vi "VelocityEstimator.vi"(8 "error in (no error)":errorcluster, 11 "Position In":dbl[](array[numeric])) -> (0 "error out":errorcluster, 3 "Vel. Out":dbl[](array[numeric]))   [LabVIEW 2018, in "Motor_ReadAng.lvlib"]
doc: "Estimate motor velocity from the motor position."
uses:
  Motor_ReadAng.lvlib
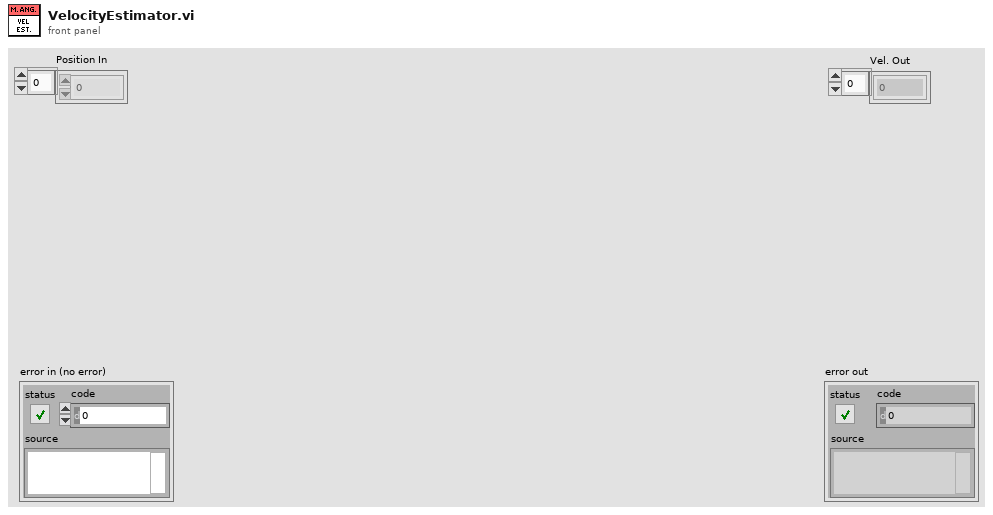
[diagram p1: front panel]
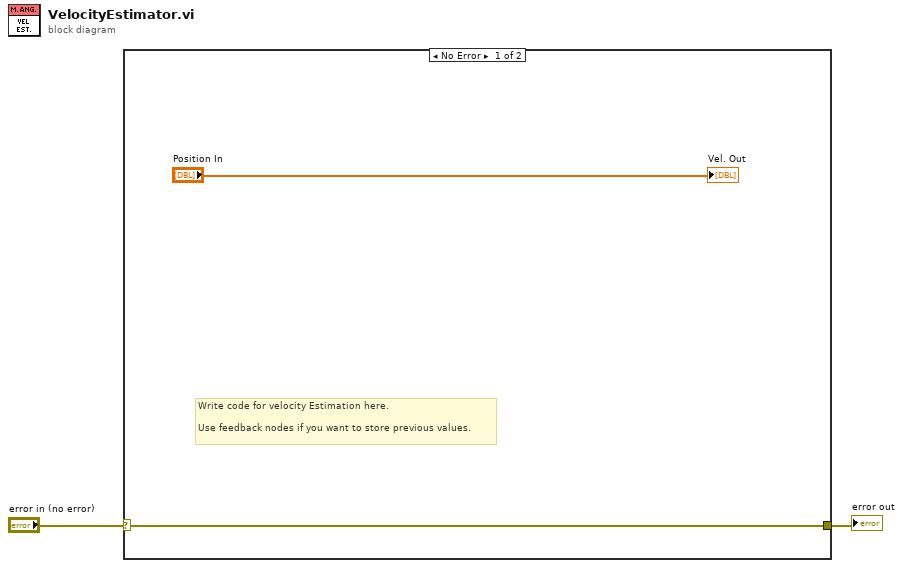
[diagram p0: block diagram]
diagram:
  n1 = case shown="No Error" "error in (no error)" {
    selector: "error in (no error)" -> [w4 w5]
    tunnel: [w4 w5] -> w1
    frame No Error {
      # "Write code for velocity Estimation here.\n\nUse feedback nodes if you want to store previous values."
      "Vel. Out" <- "Position In"
    }
    frame Error {
    }
  }
  "error out" <- w1
